vi "Ctrl.Tab, Show or Hide Tab Page.vi"(9 "Show/Hide":bool, 10 "Name":string, 11 "Tab Control":refnum<vi>) -> ()   [LabVIEW 2018]
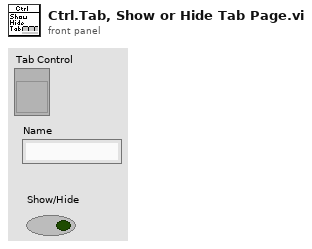
[diagram p1: front panel]
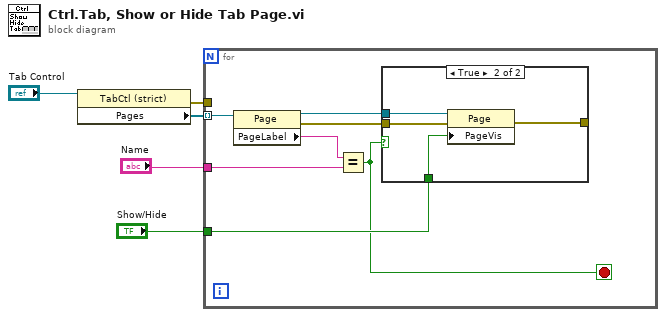
[diagram p0: block diagram]
diagram:
  n1 = property on="Property Node" class="TabCtl (strict)"(reference="Tab Control") -> (error out=w2:errorcluster, "Pages"=w5:refnum<vi>[])  [unwired: 1 in, 1 out]
  n2 = for {
    tunnel: w5 -> [w12] mode=indexing
    tunnel: "Name" -> [w9]
    tunnel: "Show/Hide" -> [w8]
    tunnel: w2 -> [_]
    stop <- w7 stop-if-true
    n3 = property class="Page"(reference=w12) -> (reference out=w10:refnum<vi>, error out=w6:errorcluster, "PageLabel"=w11:string)  [unwired: 1 in]
    n4 = Equal?(x=w11, y=w9) -> (x = y?=w7:bool)
    n5 = case shown="True" w7 {
      tunnel: w10 -> [_ w16]
      tunnel: w8 -> [_ w15]
      tunnel: w6 -> [_ w14]
      tunnel: [_ w13] -> _
      frame False {
      }
      frame True {
        n6 = property class="Page"(reference=w16, error in=w14, "PageVis"=w15) -> (error out=w13:errorcluster)  [unwired: 1 out]
      }
    }
  }
